vi "ident signals.vi"() -> ()   [LabVIEW 2015]
uses:
  <vilib>/Analysis/1siggen.llb/General Aperiodic Triangle.vi
  <vilib>/Analysis/NI_AALBase.lvlib
panel:
  out "MLS":dbl[](graph)
  out "Triangle Pattern":dbl[](graph)
  out "Gaussian WN":dbl[](graph)
  out "Uniform WN":dbl[](graph)
  out "Chirp Pattern":dbl[](graph)
  out "Sawtooth":dbl[](graph)
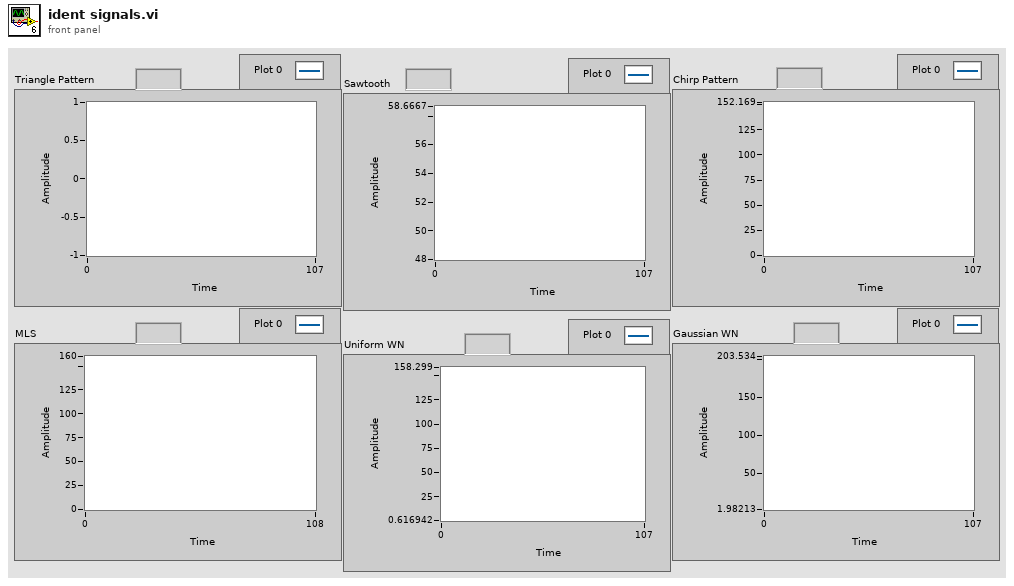
[diagram p1: front panel]
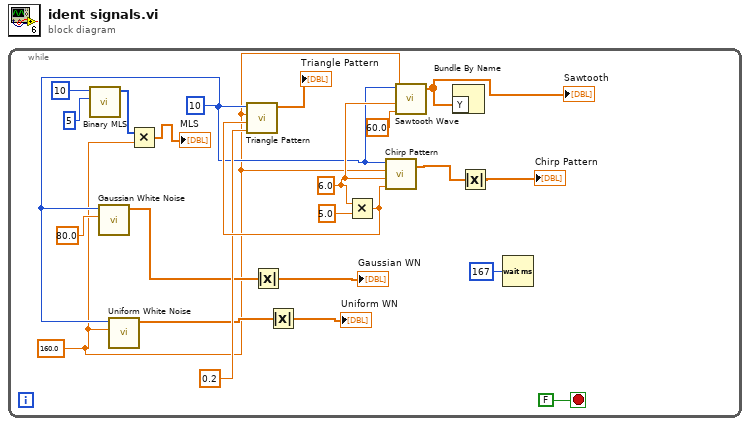
[diagram p0: block diagram]
diagram:
  n1 = while {
    stop <- FALSE stop-if-true
    w19 = 6.0 ("f1")
    w4 = 160.0 ("amplitude")
    w11 = 10 ("samples")
    n2 = call <vilib>:"Binary MLS.vi"("polynomial order"=5, "samples"=i64 10) -> ("mls sequence"=w3:u8[])  [unwired: 8 in, 1 out]
    n3 = call <vilib>:"Gaussian White Noise.vi"("standard deviation"=80.0, "samples"=w11) -> ("Gaussian noise pattern"=w6:dbl[])  [unwired: 8 in, 1 out]
    n4 = call <vilib>:"Uniform White Noise.vi"("amplitude"=w4, "samples"=w11) -> ("uniform white noise"=w5:dbl[])  [unwired: 8 in, 1 out]
    n5 = Multiply(x=w3, y=w4) -> (x*y=→"MLS":dbl[])
    n6 = Absolute Value(x=w6) -> (abs(x)=→"Gaussian WN":dbl[])
    n7 = Absolute Value(x=w5) -> (abs(x)=→"Uniform WN":dbl[])
    n8 = Multiply(x=w19, y=5.0) -> (x*y=w14:dbl)
    n9 = call <vilib>:"Triangle Pattern.vi"("delta t (s)"=0.2, "delay (s)"=w14, "amplitude"=w4, "samples"=w11) -> ("Triangle Pattern"=→"Triangle Pattern":dbl[])  [unwired: 6 in, 1 out]
    n10 = call <vilib>:"Chirp Pattern.vi"("f2"=w14, "f1"=w19, "amplitude"=w4, "samples"=w11) -> ("Chirp Pattern"=w10:dbl[])  [unwired: 1 out]
    n11 = call <vilib>:"Sawtooth Wave.vi"("samples"=w11, "amplitude"=w4, "frequency"=w19, "phase in"=60.0) -> ("sawtooth wave"=w18:dbl[])  [unwired: 1 in, 2 out]
    "Sawtooth" <- w18
    n12 = Bundle By Name("Y"=w18) -> ()  [unwired: 1 in, 1 out]
    n13 = Absolute Value(x=w10) -> (abs(x)=→"Chirp Pattern":dbl[])
    n14 = Wait (ms)(milliseconds to wait=u32 167) -> ()  [unwired: 1 out]
  }
